vi "Set DO Test.vi"(0 "Data in":cluster{"DO":bool}, 7 "DO":bool) -> (4 "Data Out":cluster{"DO":bool})   [LabVIEW 2019]
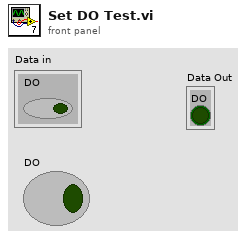
[diagram p1: front panel]
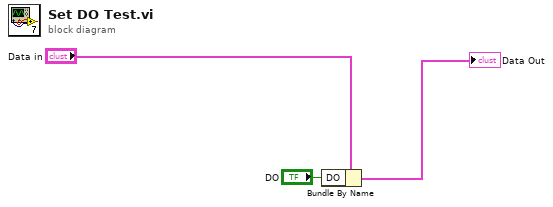
[diagram p0: block diagram]
diagram:
  n1 = Bundle By Name(cluster="Data in", "DO"="DO") -> (→"Data Out":cluster{"DO":bool})
